vi "Preview.vi"(8 "error in (no error)":errorcluster, 10 "collect dependencies? (F)":bool, 11 "Build in":refnum<class "NI_AB_API_RESTful.lvclass">) -> (0 "error out":errorcluster, 1 "Dependencies":T1[](array[typedef]), 2 "GeneratedFiles":path[](array[path]), 3 "Build out":refnum<class "NI_AB_API_RESTful.lvclass">)   [LabVIEW 2020, in "NI_AB_API_RESTful.lvclass"]
uses:
  <vilib>/AppBuilder/AB_API/RESTful/NI_AB_API_RESTful.lvclass
  <vilib>/AppBuilder/AB_API/RESTful/NI_AB_API_RESTful.lvclass/NI_AB_API_RESTful.ctl
  <vilib>/AppBuilder/AB_API/Targetfile/NI_AB_API_Targetfile.lvclass
  <vilib>/Utility/lvfile.llb/LVFileType.ctl
  <vilib>/Utility/lvfile.llb/NI_FileType.lvlib
  <vilib>/AppBuilder/AB_Dependency.ctl
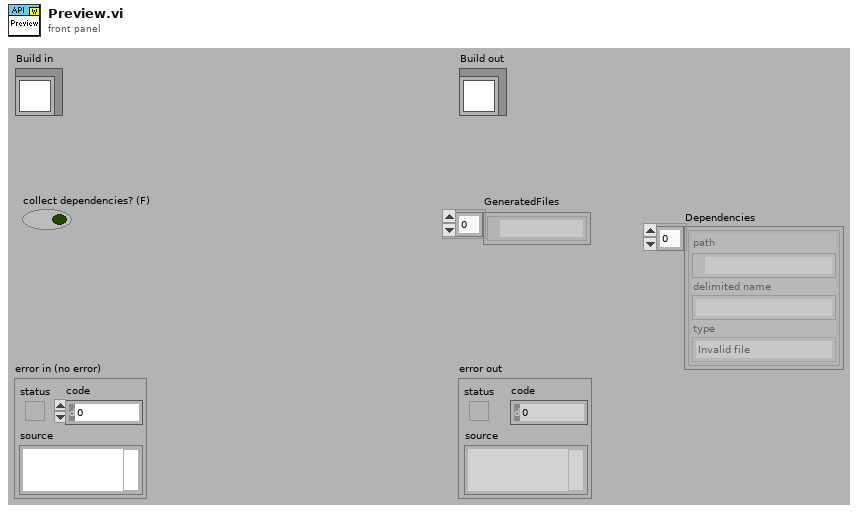
[diagram p1: front panel]
types:
  T1 = typedef "AB_Dependency.ctl" = cluster{"path":path, "delimited name":string, "type":T2}
  T2 = typedef "NI_FileType.lvlib/LVFileType.ctl" = enum32{"Invalid file", "Unknown type", "Instrument", "Control", "Polymorphic VI", "Project", "Library", "LVClass", "XControl", "XNode", "Shared library", ".NET assembly", "ActiveX interface", "CIN", "Run-time menu", "Palette menu", "Help file", "LLB", "XNode Edit Dependency", "Class Private Data Control", "Statechart", "MathScript .m file", "Ladder Diagram", "LVLibp", "XNode Build Dependency"}
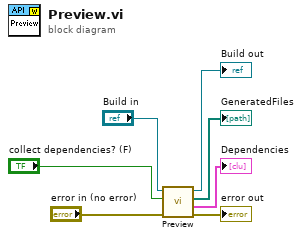
[diagram p0: block diagram]
diagram:
  n1 = call-parent "Preview.vi"("error in (no error)"="error in (no error)", "collect dependencies? (F)"="collect dependencies? (F)", "Build in"="Build in") -> ("error out"=→"error out":errorcluster, "Dependencies"=→"Dependencies":T1[], "GeneratedFiles"=→"GeneratedFiles":path[], "Build out"=→"Build out":refnum<class "NI_AB_API_RESTful.lvclass">)  [unwired: 5 in]
